vi "lowerLimit.vi"(10 "Min":dbl=-40.0, 11 "data":dbl[][](array[numeric])=[[0.0, -50.0], [-10.0, -20.0], [-70.0, -10.0]]) -> (3 "output":dbl[][](array[numeric]))   [LabVIEW 2015]
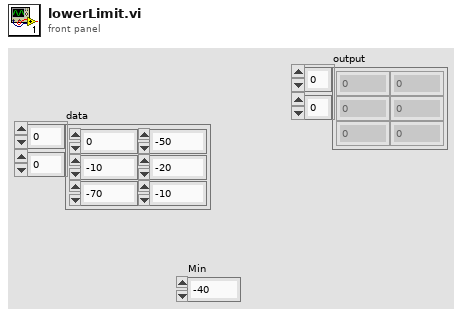
[diagram p1: front panel]
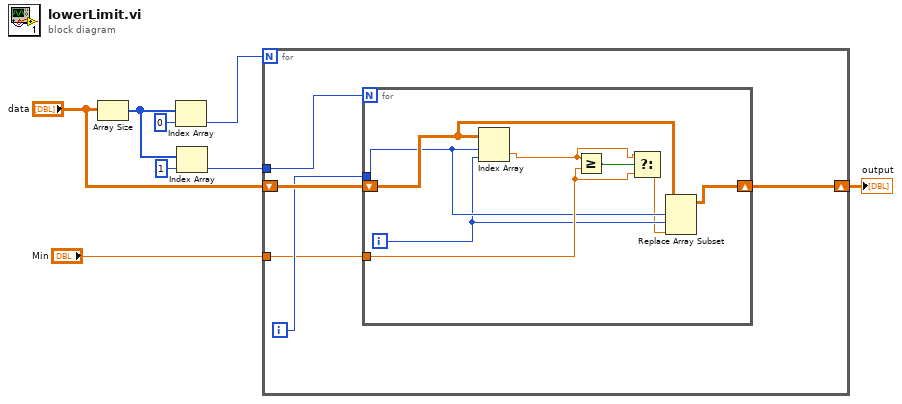
[diagram p0: block diagram]
diagram:
  n1 = Array Size(array="data") -> (size(s)=w7:i32[])
  n2 = Index Array(array=w7, index=0) -> (element=w5:i32)
  n3 = Index Array(array=w7, index=1) -> (element=w4:i32)
  n4 = for {
    N: w5 -> [_]
    tunnel: w4 -> [w13]
    shift-right: [w9] -> w1
    shift-left: "data" -> [w12]
    tunnel: "Min" -> [w10]
    i -> [w11]
    n5 = for {
      N: w13 -> [_]
      shift-right: [w14] -> w9
      shift-left: w12 -> [w18]
      tunnel: w11 -> [w17]
      tunnel: w10 -> [w19]
      i -> [w16]
      n6 = Index Array(array=w18, index (row)=w17, index (col)=w16) -> (element=w20:dbl)
      n7 = Greater Or Equal?(x=w20, y=w19) -> (x >= y?=w21:bool)
      n8 = Select(t=w20, s=w21, f=w19) -> (s? t:f=w15:dbl)
      n9 = Replace Array Subset(array=w18, new element=w15, index (row)=w17, index (col)=w16) -> (w14:dbl[][])
    }
  }
  "output" <- w1
